vi "SPD.QE Tune Phese and Get Count Rate.vi"(7 "SPD.QE Strobe_Phase Tune Limits":T1, 8 "Error In":errorcluster, 10 "Num of FreqC Meas":i32, 11 "SPD.Stand Ctrl in":T2 {"spdDeviceSession"."hidSPD.Sturtup Values"."HV_bias" format="%#_6p, V"; "spdDeviceSession"."hidSPD.Sturtup Values"."TSet" format="%#_6p, DegC"; "spdDeviceSession"."hidSPD.Controller"."HV_bias" format="%#_6p, V"; "spdDeviceSession"."hidSPD.Controller"."TSet" format="%#_6p, DegC"}) -> (0 "Error Out":errorcluster, 1 "Count Sigma":dbl, 2 "Count Rate":dbl, 3 "SPD.Stand Ctrl out":T2 {"spdDeviceSession"."hidSPD.Sturtup Values"."HV_bias" format="%#_6p, V"; "spdDeviceSession"."hidSPD.Sturtup Values"."TSet" format="%#_6p, DegC"; "spdDeviceSession"."hidSPD.Controller"."HV_bias" format="%#_6p, V"; "spdDeviceSession"."hidSPD.Controller"."TSet" format="%#_6p, DegC"})   [LabVIEW 2018]
uses:
  typedefs/SPD.Stand Ctrl.ctl
  Instruments/SPD HID Interface/hidSPDLibForLabView/LibVIs/hidSPD Controls/hidSPD Device Session.ctl
  Instruments/SPD HID Interface/hidSPDLibForLabView/LibVIs/hidSPD Controls/hidSPD Controller.ctl
  Instruments/SPD HID Interface/hidSPDLibForLabView/LibVIs/hidSPD Controls/hidSPD SPD Type.ctl
  Instruments/KC705 DevBoard/typedefs/DevB.Session.ctl
  Instruments/KeySight 53230A/typedefs/FreqC.Session.ctl
  Instruments/KeySight 8164B/KeySight 8164B LAN InstrLib/typedefs/KeySight 8164B control.ctl
  Instruments/LeCroy SDA830/typedefs/LeCroy.Session.ctl
  typedefs/SPD.Events.ctl
  ConfigFile/SPD.Config File ctrl.ctl
  <vilib>/Utility/config.llb/Config Data RefNum.ctl
  typedefs/SPD.Meas Result.ctl
  typedefs/SPD.Queues.ctl
  typedefs/SPD.Stand state.ctl
  typedefs/SPD.QE Strobe_Phase Tune Limits.ctl
  Instruments/KeySight 8164B/KeySight 8164B LAN InstrLib.lvlib
  <vilib>/Utility/config.llb/NI_LVConfig.lvlib
  Instruments/SPD HID Interface/hidSPDLibForLabView/hidSPDLibForLabView.lvlib
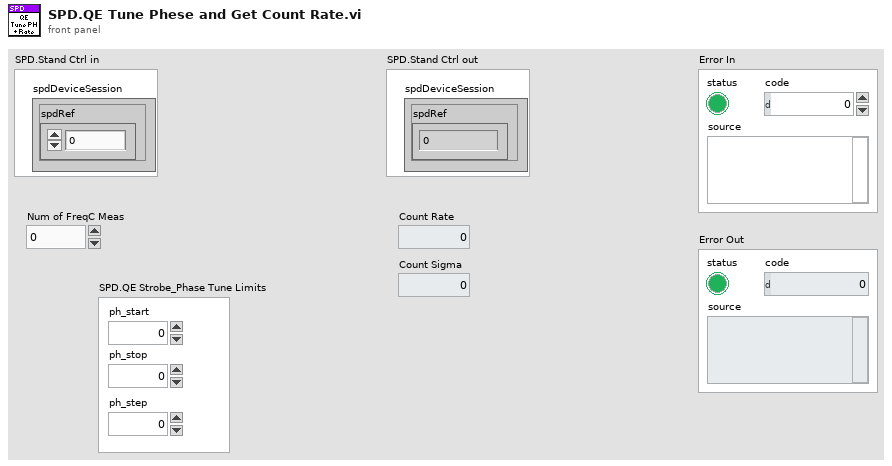
[diagram p1: front panel]
types:
  T1 = typedef "SPD.QE Strobe_Phase Tune Limits.ctl" = cluster{"ph_start":i32, "ph_stop":i32, "ph_step":i32}
  T2 = typedef "SPD.Stand Ctrl.ctl" = cluster{"spdDeviceSession":T3, "DevBSession":T6, "FreqCSession":T7, "8164BSession":T8, "LeCroySession":T9, "Events":T10, "configFile":T11, "SPD.Result":T13, "SPD.Queues":T14, "Console":refnum<vi>}
  T3 = typedef "hidSPDLibForLabView.lvlib/hidSPD Device Session.ctl" = cluster{"spdRef":u64, "connected":bool, "spdName":string, "hidSPD.Controller":T4, "hidSPD.Sturtup Values":T4, "SPD Type":T5}
  T4 = typedef "hidSPDLibForLabView.lvlib/hidSPD Controller.ctl" = cluster{"TSet":sgl, "HV_bias":sgl, "DDS_stb_code":u16}
  T5 = typedef "hidSPDLibForLabView.lvlib/hidSPD SPD Type.ctl" = enum16{"Free Run", "Strobe"}
  T6 = typedef "DevB.Session.ctl" = cluster{"DevBRef":refnum<visa-resource-name>, "connected":bool}
  T7 = typedef "FreqC.Session.ctl" = cluster{"FreqCRef":refnum<visa-resource-name>, "timeout":dbl, "Gate":dbl, "connected":bool}
  T8 = typedef "KeySight 8164B LAN InstrLib.lvlib/KeySight 8164B control.ctl" = cluster{"Connection ID":refnum<k5>, "Connected":bool, "Info":string, "Slots Info":string[]}
  T9 = typedef "LeCroy.Session.ctl" = cluster{"LeCroySession":refnum<visa-resource-name>, "connected":bool}
  T10 = typedef "SPD.Events.ctl" = cluster{"DCRTest":refnum<user-event>, "Stop":refnum<user-event>}
  T11 = typedef "SPD.Config File ctrl.ctl" = cluster{"configFile ref":T12, "configFile path":path, "equipmentFile ref":T12}
  T12 = typedef "NI_LVConfig.lvlib/Config Data RefNum.ctl" = refnum<k1>
  T13 = typedef "SPD.Meas Result.ctl" = cluster{"HV_Bias":dbl[][][], "Stb_code":dbl[], "Temprature":dbl[], "Data":dbl[][][][], "DateTime":string}
  T14 = typedef "SPD.Queues.ctl" = cluster{"state queue":refnum<queue>}
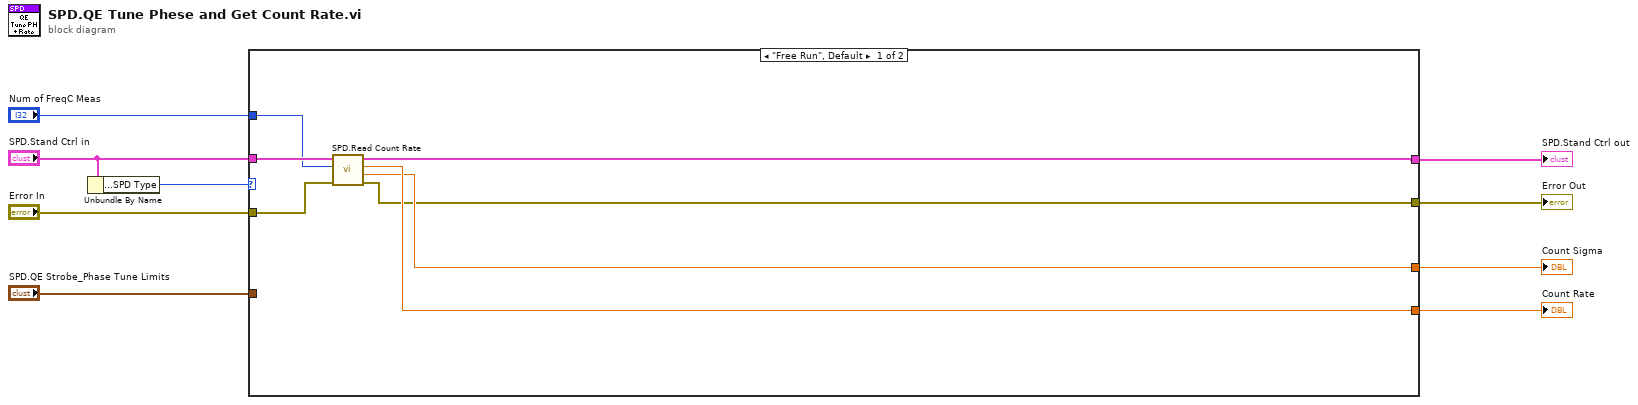
[diagram p0: block diagram]
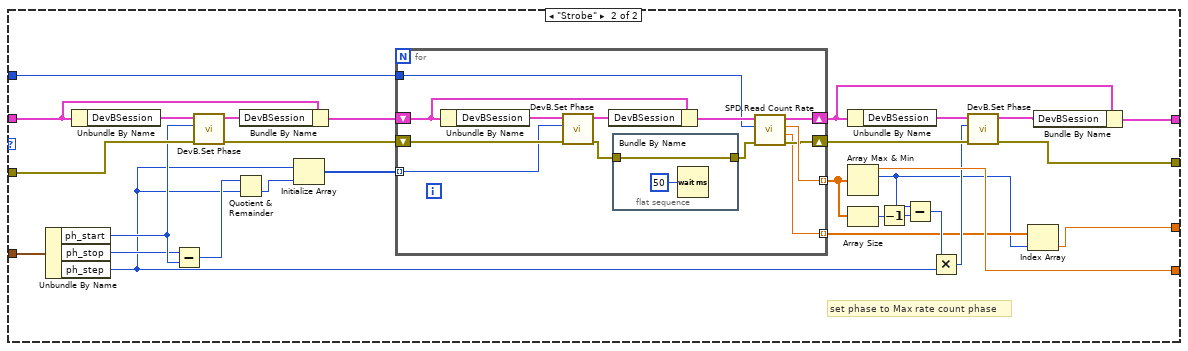
[diagram p2: hidden frame]
diagram:
  n1 = Unbundle By Name("SPD.Stand Ctrl in") -> ("spdDeviceSession.SPD Type"=w1:T5)
  n2 = case shown="\"Free Run\", Default" w1 {
    tunnel: "Num of FreqC Meas" -> [w14 w42]
    tunnel: [w13 w41] -> w8
    tunnel: "SPD.Stand Ctrl in" -> [w16 w35]
    tunnel: "Error In" -> [w15 w34]
    tunnel: [w10 w25] -> w6
    tunnel: [w11 w24] -> w5
    tunnel: "SPD.QE Strobe_Phase Tune Limits" -> [_ w23]
    tunnel: [w12 w17] -> w3
    frame "Free Run", Default {
      n3 = call "SPD.Read Count Rate.vi"("Error In"=w15, "Num of Meas"=w14, "SPD.Stand Ctrl in"=w16) -> ("Error Out"=w11:errorcluster, "Count sigma"=w12:dbl, "Count"=w13:dbl, "SPD.Stand Ctrl out"=w10:T2)  [unwired: 5 in]
    }
    frame "Strobe" {
      # "set phase to Max rate count phase"
      n4 = Unbundle By Name(w23) -> ("ph_start"=w22:i32, "ph_stop"=w21:i32, "ph_step"=w20:i32)
      n5 = Unbundle By Name(w35) -> ("DevBSession"=w37:T6)
      n6 = Subtract(x=w21, y=w22) -> (x-y=w45:i32)
      n7 = call "DevB.Set Phase.vi"("error in (no error)"=w34, "Phase"=w22, "DevB Session in"=w37) -> ("error out"=w32:errorcluster, "DevB Session out"=w36:T6)  [unwired: 7 in]
      n8 = Quotient & Remainder(x=w45, y=w20) -> (floor(x/y)=w44:i32)  [unwired: 1 out]
      n9 = Bundle By Name(cluster=w35, "DevBSession"=w36) -> (w33:T2)
      n10 = Initialize Array(w20, w44) -> (w43:i32[])
      n11 = for {
        tunnel: w43 -> [w47] mode=indexing
        shift-right: [w49] -> w31
        shift-left: w32 -> [w55]
        tunnel: w42 -> [w53]
        tunnel: [w50] -> w30 mode=indexing
        shift-right: [w48] -> w40
        shift-left: w33 -> [w58]
        tunnel: [w46] -> w19 mode=indexing
        n12 = Unbundle By Name(w58) -> ("DevBSession"=w57:T6)
        n13 = call "DevB.Set Phase.vi"("error in (no error)"=w55, "Phase"=w47, "DevB Session in"=w57) -> ("error out"=w52:errorcluster, "DevB Session out"=w56:T6)  [unwired: 7 in]
        n14 = Bundle By Name(cluster=w58, "DevBSession"=w56) -> (w54:T2)
        n15 = flat-sequence {
          tunnel: w52 -> [w60]
          tunnel: [w60] -> w51
          frame #0 {
            n16 = Wait (ms)(milliseconds to wait=u32 50) -> ()  [unwired: 1 out]
          }
        }
        n17 = call "SPD.Read Count Rate.vi"("Error In"=w51, "Num of Meas"=w53, "SPD.Stand Ctrl in"=w54) -> ("Error Out"=w49:errorcluster, "Count sigma"=w46:dbl, "Count"=w50:dbl, "SPD.Stand Ctrl out"=w48:T2)  [unwired: 5 in]
      }
      n18 = Unbundle By Name(w40) -> ("DevBSession"=w39:T6)
      n19 = Array Max & Min(array=w30) -> (max value=w41:dbl, max index (indices)=w18:i32)  [unwired: 2 out]
      n20 = Array Size(array=w30) -> (size(s)=w29:i32)
      n21 = Decrement(x=w29) -> (x-1=w28:i32)
      n22 = Subtract(x=w18, y=w28) -> (x-y=w27:i32)
      n23 = Multiply(x=w27, y=w20) -> (x*y=w26:i32)
      n24 = call "DevB.Set Phase.vi"("error in (no error)"=w31, "Phase"=w26, "DevB Session in"=w39) -> ("error out"=w24:errorcluster, "DevB Session out"=w38:T6)  [unwired: 7 in]
      n25 = Index Array(array=w19, index=w18) -> (element=w17:dbl)
      n26 = Bundle By Name(cluster=w40, "DevBSession"=w38) -> (w25:T2)
    }
  }
  "SPD.Stand Ctrl out" <- w6
  "Error Out" <- w5
  "Count Rate" <- w8
  "Count Sigma" <- w3
